vi "ezAFM Practice 1.5.vi"() -> ()   [LabVIEW 2015]
uses:
  D:/LabVIEW for ezAFM/LV-PGC 2019-05a/Special Equipment/ezAFM/NMI Integration Code/ezCommander.dll
  LabVIEW for ezAFM/LV-PGC 2019-05a/Special Equipment/ezAFM/NMI Integration Code/ezCommander.dll
  <vilib>/userdefined/High Color/IMAQdx.ctl
  LabVIEW for ezAFM/LV-PGC 2019-05a/Universal vi's/Global Variables/Globals-EasyAFM.vi
  Globals.vi
  <vilib>/vision/driver/NI_Vision_Acquisition_Software.lvlib
panel:
  out "Index":dbl
  out "Direction":dbl
  out "Searching":bool
  out "Crosshair Found?":bool
  in  "Search":bool
  out "Total Steps":dbl
  out "Current Steps":dbl
  in  "Camera":enum32{"ezAFM Camera"}(tab)
  out "ezAFM Camera":T1(plugin-control)
  out "Currently Scanning":string
  in  "Enable Automatic Repositioning?":bool
  in  "Main Menu":enum32{"Navigation", "Scanning"}(tab)
  in  "APPROACH":bool
  in  "RETRACT":bool
  in  "Step Size":dbl
  out "Angle":dbl
  in  "THETA":bool
  in  "MOVE2CROSSHAIR":bool
  in  "Current Crosshair":string(combo)="00 | 01"
  in  "Target Crosshair":string(combo)="00 | 01"
  in  "Motor Speed":u16(ring)=30000 items=["SLOW"=3300, "MEDIUM"=30000, "FAST"=65000]
  in  "Navigation Buttons":T2
  in  "SEARCH":bool
  in  "Image Resolution":u16(ring)=256 items=["32"=32, "64"=64, "128"=128, "256"=256, "512"=512, "1024"=1024, "2048"=2048]
  in  "SELECT CONNECTIONS":bool
  in  "BEGIN AUTOMATED IMAGING":bool
  out "Connections":string[](array[string])
  in  "Indicators":enum32{"Indicators"}(tab)
  out "XYZ Motor Position":dbl[](array[numeric]) format="%#_4f"
  out "ezAFM Status":dbl
  out "Approaching":bool
  out "ezAFM Connected":bool
  out "Retracting":bool
  out "Scanning":bool
  out "Tip Approached?":bool
  in  "RESET":bool
  out "XY Position":dbl[](array[numeric])
  in  "QUIT":bool
  # "Use Arrow Keys to manually\nmove the XY Motor"
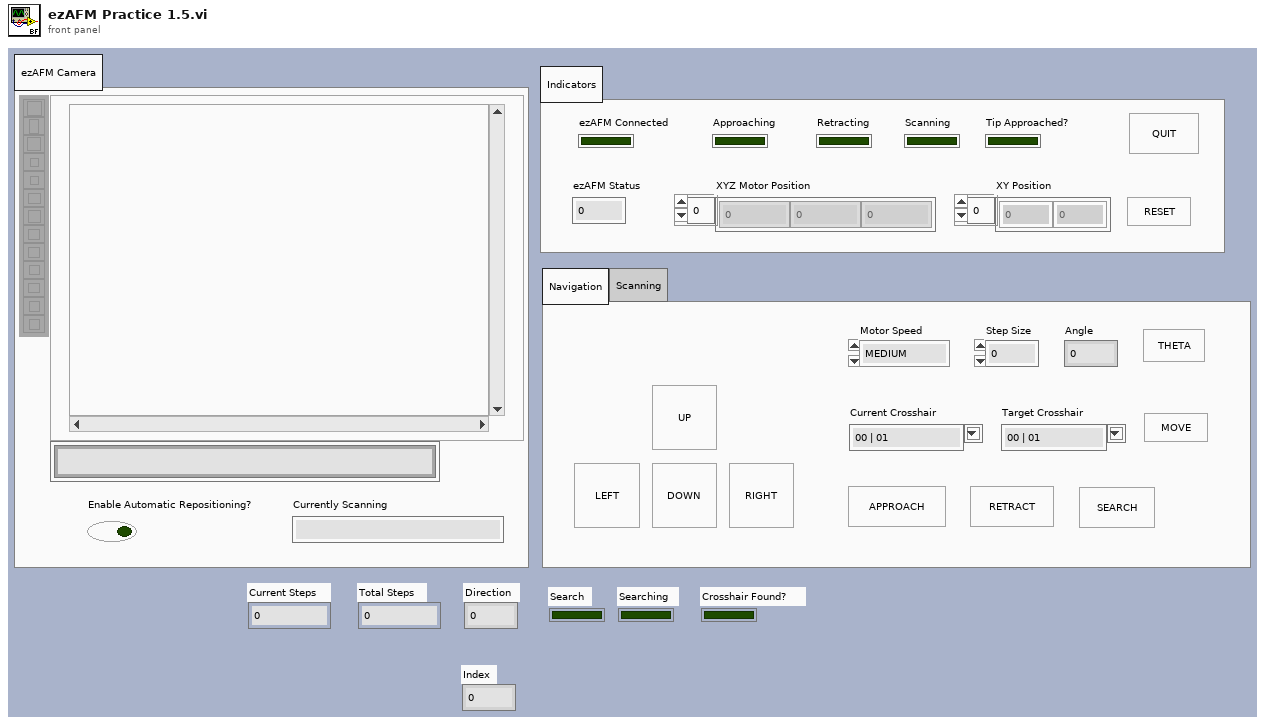
[diagram p1: front panel]
types:
  T1 = typedef "IMAQ Image.ctl" = refnum<image>
  T2 = cluster{"UP":bool, "DOWN":bool, "LEFT":bool, "RIGHT":bool}
  T3 = typedef "IMAQdx.ctl" = refnum<k21>
  T4 = typedef "Image Type" = u32
  T5 = typedef "eventvkey.ctl" = enum16{"ASCII", "Enter", "Return", "Shift", "Ctrl", "Alt", "Cmd", "Opt", "Caps", "NumLock", "Clear", "Break", "Up", "Down", "Left", "Right", "Insert", "Delete", "Home", "End", "PageUp", "PageDown", "Escape", "Help", "Pause", "ScrollLock", "F1", "F2", "F3", "F4", "F5", "F6", "F7", "F8", "F9", "F10", "F11", "F12", "F13", "F14", "F15", "F16", "F17", "F18", "F19", "F20", "F21", "F22", "F23", "F24", "Play", "VolumeUp", "VolumeDown", "Mute", "Two Byte Char"}
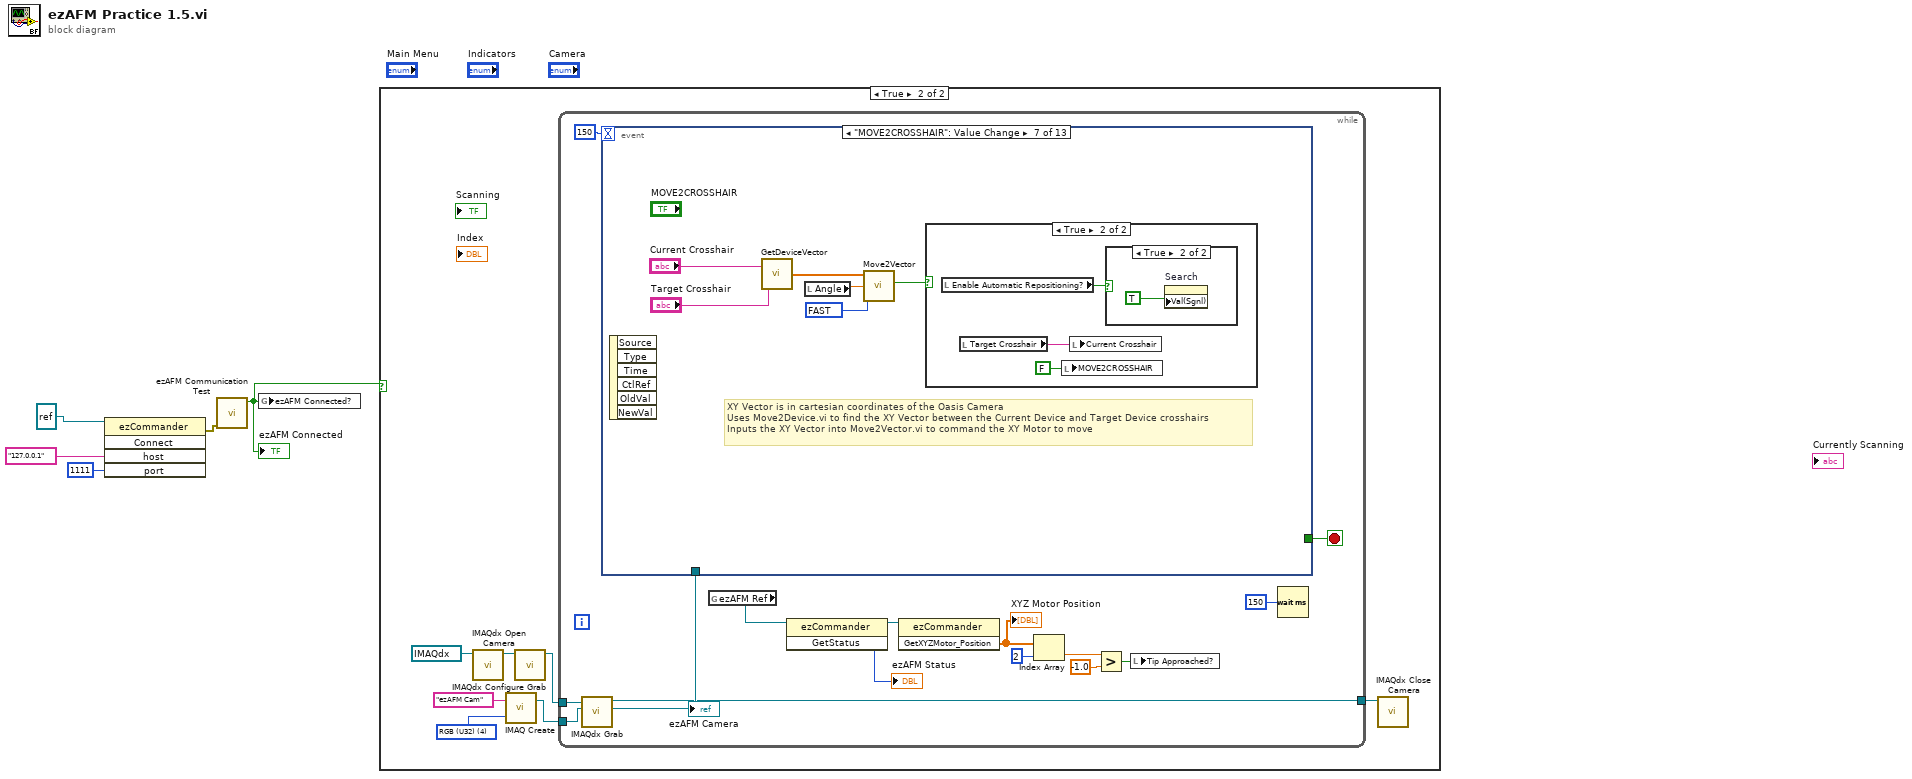
[diagram p0: block diagram]
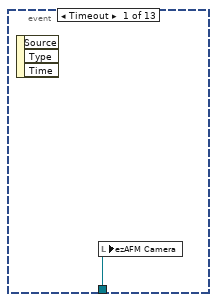
[diagram p3: hidden frame]
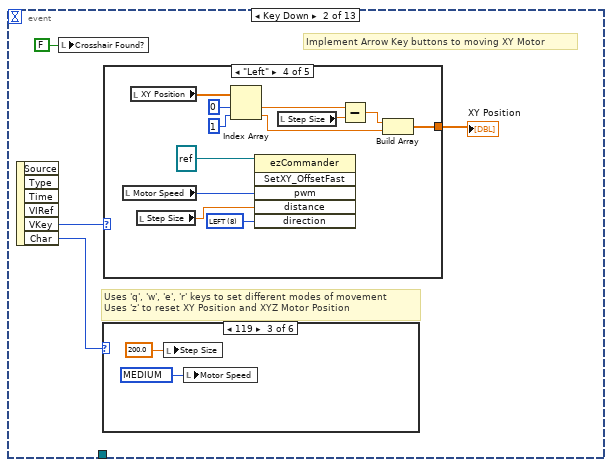
[diagram p4: hidden frame]
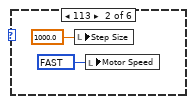
[diagram p6: hidden frame]
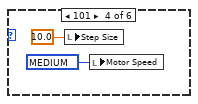
[diagram p7: hidden frame]
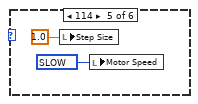
[diagram p8: hidden frame]
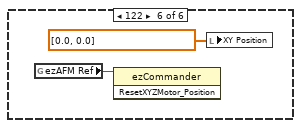
[diagram p9: hidden frame]
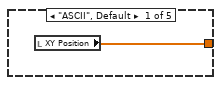
[diagram p10: hidden frame]
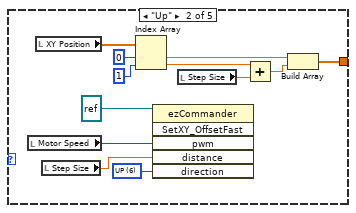
[diagram p11: hidden frame]
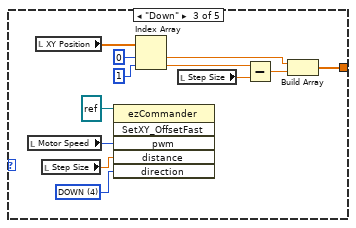
[diagram p12: hidden frame]
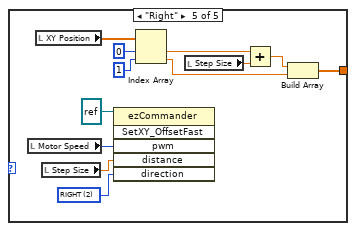
[diagram p13: hidden frame]
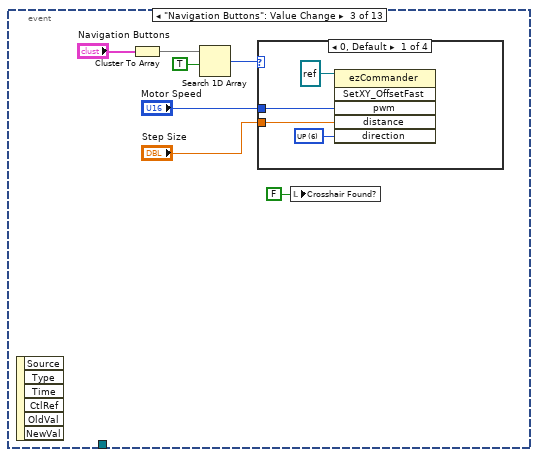
[diagram p14: hidden frame]
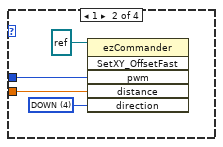
[diagram p15: hidden frame]
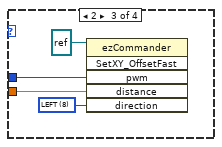
[diagram p16: hidden frame]
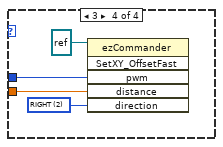
[diagram p17: hidden frame]
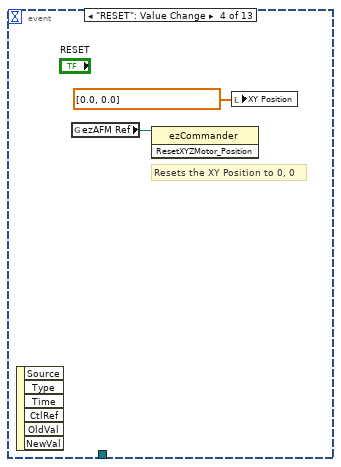
[diagram p18: hidden frame]
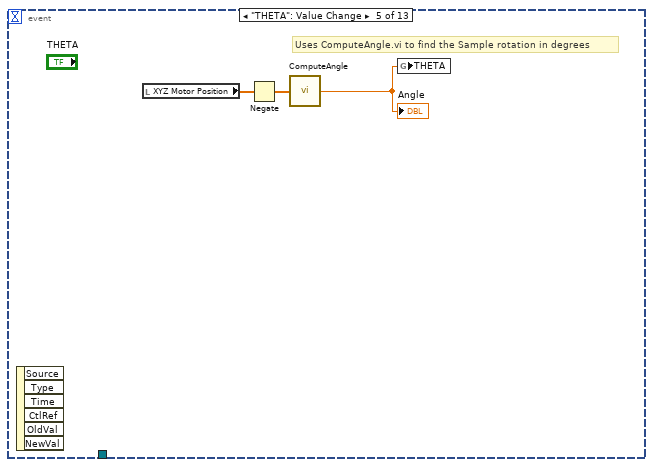
[diagram p19: hidden frame]
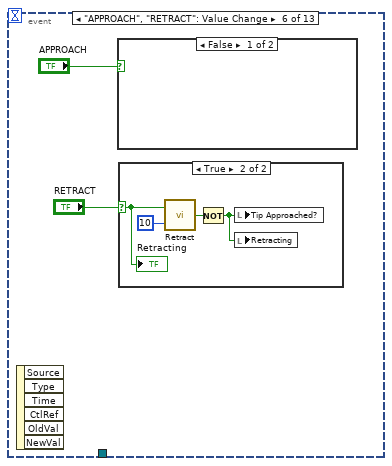
[diagram p20: hidden frame]
diagram:
  n1 = invoke class="ezCommander" method="Connect"(reference=refnum<k24> refnum ("ezAFM Ref"), "host"="127.0.0.1", "port"=1111) -> (error out=w4:errorcluster)  [unwired: 2 in, 4 out]
  n2 = call "ezAFM Communication Test.vi"("error in"=w4) -> ("ezAFM COM status"=w1:bool)  [unwired: 3 in, 3 out]
  "ezAFM Connected" <- w1
  n3 = global write "Globals.vi" "ezAFM Connected?"(w1) -> ()
  n4 = case shown="True" w1 {
    frame False {
    }
    frame True {
      w8 = T4 4 items=["Grayscale (U8)", "Grayscale (I16)", "Grayscale (SGL)", "Complex (CSG)", "RGB (U32)", "HSL (U32)", "RGB (U64)", "Grayscale (U16)"] ("Image Type")
      n5 = call <vilib>:"IMAQdx Open Camera.vi"("Session In"=T3 "cam5") -> ("Session Out"=w10:T3)  [unwired: 9 in, 1 out]
      n6 = call "IMAQ Create"("Image Name"="ezAFM Cam", "Image Type"=w8) -> ("New Image"=w9:T1)  [unwired: 3 in, 1 out]
      n7 = call <vilib>:"IMAQdx Configure Grab.vi"("Session In"=w10) -> ("Session Out"=w7:T3)  [unwired: 9 in, 1 out]
      n8 = while {
        tunnel: w9 -> [w26]
        tunnel: w7 -> [w25]
        tunnel: [w15] -> w6
        stop <- w14 stop-if-true
        n9 = call <vilib>:"IMAQdx Grab.vi"("Image In"=w26, "Session In"=w25) -> ("Image Out"=w16:T1, "Session Out"=w15:T3)  [unwired: 2 in, 6 out]
        "ezAFM Camera" <- w16
        n10 = event shown="[6] \"MOVE2CROSSHAIR\": Value Change" {
          selector: _ -> [_ _ _ _ _ _ _ _ _ _ _ _ _]
          dyn-events: _ -> [_ _ _ _ _ _ _ _ _ _ _ _ _]
          timeout: 150 -> [_ _ _ _ _ _ _ _ _ _ _ _ _]
          tunnel: [_ _ _ _ _ _ _ _ _ _ _ _ "QUIT"] -> w14
          tunnel: w16 -> [w28 _ _ _ _ _ _ _ _ _ w173 _ _]
          event Timeout {
            n11 = event-data() -> ()  [unwired: 1 in, 3 out]
            n12 = local write "ezAFM Camera"(w28) -> ()
          }
          event Key Down {
            # "Uses 'q', 'w', 'e', 'r' keys to set different modes of movement\nUses 'z' to reset XY Position and XYZ Motor Position"
            # "Implement Arrow Key buttons to moving XY Motor"
            n13 = event-data() -> ("VKey"=w30:T5, "Char"=w31:i16)  [unwired: 1 in, 4 out]
            n14 = local write "Crosshair Found?"(FALSE ("Crosshair Found?")) -> ()
            n15 = case shown="119" w31 {
              frame 0, Default {
              }
              frame 113 {
                w33 = u16 65000 items=["SLOW"=3300, "MEDIUM"=30000, "FAST"=65000] ("Motor Speed")
                n16 = local write "Step Size"(1000.0 ("Step Size")) -> ()
                n17 = local write "Motor Speed"(w33) -> ()
              }
              frame 119 {
                w35 = u16 30000 items=["SLOW"=3300, "MEDIUM"=30000, "FAST"=65000] ("Motor Speed")
                n18 = local write "Step Size"(200.0 ("Step Size")) -> ()
                n19 = local write "Motor Speed"(w35) -> ()
              }
              frame 101 {
                w37 = u16 30000 items=["SLOW"=3300, "MEDIUM"=30000, "FAST"=65000] ("Motor Speed")
                n20 = local write "Step Size"(10.0 ("Step Size")) -> ()
                n21 = local write "Motor Speed"(w37) -> ()
              }
              frame 114 {
                w39 = u16 3300 items=["SLOW"=3300, "MEDIUM"=30000, "FAST"=65000] ("Motor Speed")
                n22 = local write "Step Size"(1.0 ("Step Size")) -> ()
                n23 = local write "Motor Speed"(w39) -> ()
              }
              frame 122 {
                n24 = global read "Globals-EasyAFM.vi" "ezAFM Ref"() -> (w41:refnum<k24>)
                n25 = invoke class="ezCommander" method="ResetXYZMotor_Position"(reference=w41) -> ()  [unwired: 2 in, 3 out]
                n26 = local write "XY Position"(dbl[] [0.0, 0.0] ("XY Position")) -> ()
              }
            }
            n27 = case shown="\"Left\"" w30 {
              tunnel: [w43 w45 w56 w68 w80] -> w32
              frame "ASCII", Default {
                n28 = local read "XY Position"() -> (w43:dbl[])
              }
              frame "Up" {
                w54 = u16 6 items=["UP"=6, "DOWN"=4, "LEFT"=8, "RIGHT"=2]
                n29 = local read "Motor Speed"() -> (w53:u16)
                n30 = local read "XY Position"() -> (w51:dbl[])
                n31 = local read "Step Size"() -> (w52:dbl)
                n32 = Index Array(array=w51, index #1=0 ("index"), index #2=1 ("index")) -> (element #1=w47:dbl, element #2=w44:dbl)
                n33 = invoke class="ezCommander" method="SetXY_OffsetFast"(reference=refnum<k24> refnum ("ezAFM Ref"), "pwm"=w53, "distance"=w52, "direction"=w54) -> ()  [unwired: 2 in, 6 out]
                n34 = local read "Step Size"() -> (w48:dbl)
                n35 = Add(x=w44, y=w48) -> (x+y=w46:dbl)
                n36 = Build Array(w47, w46) -> (w45:dbl[])
              }
              frame "Down" {
                w64 = u16 4 items=["UP"=6, "DOWN"=4, "LEFT"=8, "RIGHT"=2]
                n37 = local read "Motor Speed"() -> (w66:u16)
                n38 = local read "XY Position"() -> (w58:dbl[])
                n39 = local read "Step Size"() -> (w65:dbl)
                n40 = invoke class="ezCommander" method="SetXY_OffsetFast"(reference=refnum<k24> refnum ("ezAFM Ref"), "pwm"=w66, "distance"=w65, "direction"=w64) -> ()  [unwired: 2 in, 6 out]
                n41 = Index Array(array=w58, index #1=0 ("index"), index #2=1 ("index")) -> (element #1=w60:dbl, element #2=w61:dbl)
                n42 = local read "Step Size"() -> (w57:dbl)
                n43 = Subtract(x=w61, y=w57) -> (x-y=w59:dbl)
                n44 = Build Array(w60, w59) -> (w56:dbl[])
              }
              frame "Left" {
                w78 = u16 8 items=["UP"=6, "DOWN"=4, "LEFT"=8, "RIGHT"=2]
                n45 = local read "Motor Speed"() -> (w76:u16)
                n46 = local read "XY Position"() -> (w72:dbl[])
                n47 = local read "Step Size"() -> (w77:dbl)
                n48 = Index Array(array=w72, index #1=0 ("index"), index #2=1 ("index")) -> (element #1=w71:dbl, element #2=w69:dbl)
                n49 = invoke class="ezCommander" method="SetXY_OffsetFast"(reference=refnum<k24> refnum ("ezAFM Ref"), "pwm"=w76, "distance"=w77, "direction"=w78) -> ()  [unwired: 2 in, 6 out]
                n50 = local read "Step Size"() -> (w73:dbl)
                n51 = Subtract(x=w71, y=w73) -> (x-y=w70:dbl)
                n52 = Build Array(w70, w69) -> (w68:dbl[])
              }
              frame "Right" {
                w90 = u16 2 items=["UP"=6, "DOWN"=4, "LEFT"=8, "RIGHT"=2]
                n53 = local read "Motor Speed"() -> (w89:u16)
                n54 = local read "XY Position"() -> (w85:dbl[])
                n55 = local read "Step Size"() -> (w88:dbl)
                n56 = invoke class="ezCommander" method="SetXY_OffsetFast"(reference=refnum<k24> refnum ("ezAFM Ref"), "pwm"=w89, "distance"=w88, "direction"=w90) -> ()  [unwired: 2 in, 6 out]
                n57 = Index Array(array=w85, index #1=0 ("index"), index #2=1 ("index")) -> (element #1=w83:dbl, element #2=w81:dbl)
                n58 = local read "Step Size"() -> (w84:dbl)
                n59 = Add(x=w83, y=w84) -> (x+y=w82:dbl)
                n60 = Build Array(w82, w81) -> (w80:dbl[])
              }
            }
            "XY Position" <- w32
          }
          event "Navigation Buttons": Value Change {
            n61 = event-data() -> ()  [unwired: 1 in, 6 out]
            n62 = Cluster To Array(cluster="Navigation Buttons") -> (array=w97:bool[])
            n63 = Search 1D Array(1D array=w97, element=TRUE) -> (index of element=w95:i32)  [unwired: 1 in]
            n64 = case shown="0, Default" w95 {
              tunnel: "Step Size" -> [w99 w104 w108 w112]
              tunnel: "Motor Speed" -> [w100 w103 w107 w111]
              frame 0, Default {
                w101 = u16 6 items=["UP"=6, "DOWN"=4, "LEFT"=8, "RIGHT"=2]
                n65 = invoke class="ezCommander" method="SetXY_OffsetFast"(reference=refnum<k24> refnum ("ezAFM Ref"), "pwm"=w100, "distance"=w99, "direction"=w101) -> ()  [unwired: 2 in, 6 out]
              }
              frame 1 {
                w105 = u16 4 items=["UP"=6, "DOWN"=4, "LEFT"=8, "RIGHT"=2]
                n66 = invoke class="ezCommander" method="SetXY_OffsetFast"(reference=refnum<k24> refnum ("ezAFM Ref"), "pwm"=w103, "distance"=w104, "direction"=w105) -> ()  [unwired: 2 in, 6 out]
              }
              frame 2 {
                w109 = u16 8 items=["UP"=6, "DOWN"=4, "LEFT"=8, "RIGHT"=2]
                n67 = invoke class="ezCommander" method="SetXY_OffsetFast"(reference=refnum<k24> refnum ("ezAFM Ref"), "pwm"=w107, "distance"=w108, "direction"=w109) -> ()  [unwired: 2 in, 6 out]
              }
              frame 3 {
                w113 = u16 2 items=["UP"=6, "DOWN"=4, "LEFT"=8, "RIGHT"=2]
                n68 = invoke class="ezCommander" method="SetXY_OffsetFast"(reference=refnum<k24> refnum ("ezAFM Ref"), "pwm"=w111, "distance"=w112, "direction"=w113) -> ()  [unwired: 2 in, 6 out]
              }
            }
            n69 = local write "Crosshair Found?"(FALSE ("Crosshair Found?")) -> ()
          }
          event "RESET": Value Change {
            # "Resets the XY Position to 0, 0"
            n70 = event-data() -> ()  [unwired: 1 in, 6 out]
            n71 = global read "Globals-EasyAFM.vi" "ezAFM Ref"() -> (w115:refnum<k24>)
            n72 = invoke class="ezCommander" method="ResetXYZMotor_Position"(reference=w115) -> ()  [unwired: 2 in, 3 out]
            n73 = local write "XY Position"(dbl[] [0.0, 0.0] ("XY Position")) -> ()
          }
          event "THETA": Value Change {
            # "Uses ComputeAngle.vi to find the Sample rotation in degrees"
            n74 = event-data() -> ()  [unwired: 1 in, 6 out]
            n75 = local read "XYZ Motor Position"() -> (w117:dbl[])
            n76 = Negate(x=w117) -> (-x=w118:dbl[])
            n77 = call "ComputeAngle.vi"("XY Vector"=w118) -> ("Angle"=w119:dbl)
            "Angle" <- w119
            n78 = global write "Globals.vi" "THETA"(w119) -> ()
          }
          event "APPROACH", "RETRACT": Value Change {
            n79 = event-data() -> ()  [unwired: 1 in, 6 out]
            n80 = case shown="False" "APPROACH" {
              selector: "APPROACH" -> [_ w127]
              frame False {
              }
              frame True {
                n81 = call "AutoLand&Approach.vi"("Approaching?"=w127) -> ("Finished?"=w126:bool)
                "Tip Approached?" <- w126
                n82 = Not(x=w126) -> (.not. x?=w128:bool)
                n83 = local write "Approaching"(w128) -> ()
                "Approaching" <- w127
              }
            }
            n84 = case shown="True" "RETRACT" {
              selector: "RETRACT" -> [_ w122]
              frame False {
              }
              frame True {
                n85 = call "Retract.vi"("Number of Cycles"=10, "Retracting?"=w122) -> ("Finished?"=w124:bool)
                n86 = Not(x=w124) -> (.not. x?=w123:bool)
                n87 = local write "Tip Approached?"(w123) -> ()
                n88 = local write "Retracting"(w123) -> ()
                "Retracting" <- w122
              }
            }
          }
          event "MOVE2CROSSHAIR": Value Change {
            w133 = u16 65000 items=["SLOW"=3300, "MEDIUM"=30000, "FAST"=65000] ("Motor Speed")
            # "XY Vector is in cartesian coordinates of the Oasis Camera\nUses Move2Device.vi to find the XY Vector between the Current Device and Target Device crosshairs\nInputs the XY Vector into Move2Vector.vi to command the XY Motor to move"
            n89 = event-data() -> ()  [unwired: 1 in, 6 out]
            n90 = call "GetDeviceVector.vi"("Target Device"="Target Crosshair", "Current Device"="Current Crosshair") -> ("XY Vector"=w134:dbl[])
            n91 = local read "Angle"() -> (w132:dbl)
            n92 = call "Move2Vector.vi"("Motor Speed"=w133, "Angle"=w132, "XY Vector"=w134) -> ("Finished?"=w129:bool)  [unwired: 8 in]
            n93 = case shown="True" w129 {
              frame False {
              }
              frame True {
                n94 = local read "Enable Automatic Repositioning?"() -> (w137:bool)
                n95 = local read "Target Crosshair"() -> (w136:string)
                n96 = local write "MOVE2CROSSHAIR"(FALSE) -> ()
                n97 = local write "Current Crosshair"(w136) -> ()
                n98 = case shown="True" w137 {
                  frame False {
                  }
                  frame True {
                    n99 = property on="Search" class="Bool (strict)"("Val(Sgnl)"=TRUE ("Value (Signaling)")) -> ()  [unwired: 2 in, 2 out]
                  }
                }
              }
            }
          }
          event "SELECT CONNECTIONS": Value Change {
            n100 = event-data() -> ()  [unwired: 1 in, 6 out]
            n101 = case shown="True" "SELECT CONNECTIONS" {
              frame False {
              }
              frame True {
                n102 = call "SelectConnections.vi"() -> ("Selected Connections"=→"Connections":string[])  [unwired: 1 in]
              }
            }
          }
          event "Enable Automatic Repositioning?": Value Change {
            w141 = u16 6 items=["UP"=6, "DOWN"=4, "LEFT"=8, "RIGHT"=2]
            n103 = event-data() -> ()  [unwired: 1 in, 6 out]
            "Total Steps" <- 1.0 ("Total Distance")
            "Current Steps" <- 0.0 ("Current Steps")
            "Direction" <- w141
          }
          event "BEGIN AUTOMATED IMAGING": Value Change {
            n104 = event-data() -> ("NewVal"=w144:bool)  [unwired: 1 in, 5 out]
            n105 = local read "Connections"() -> (w147:string[])
            n106 = local write "Enable Automatic Repositioning?"(w144) -> ()
            n107 = call "BuildSequence.vi"("Connections"=w147) -> ("Sequence"=w146:string[])
            n108 = for {
              tunnel: w146 -> [w149] mode=indexing
              tunnel: "Image Resolution" -> [w148]
              n109 = Search/Split String(string=w149, search string/char (-)="Scan Spot") -> (offset of match=w152:i32)  [unwired: 1 in, 2 out]
              n110 = Search/Split String(string=w149, search string/char (-)="Crosshairs") -> (offset of match=w153:i32)  [unwired: 1 in, 2 out]
              n111 = Greater Or Equal To 0?(x=w152) -> (x >= 0?=w151:bool)
              n112 = Greater Or Equal To 0?(x=w153) -> (x >= 0?=w150:bool)
              n113 = case shown="True" w150 {
                tunnel: w149 -> [_ w160]
                frame False {
                }
                frame True {
                  n114 = String Subset(string=w160, offset (0)=21, length (rest)=7 ("length (rest)")) -> (substring=w158:string)
                  n115 = String Subset(string=w160, offset (0)=10, length (rest)=7 ("length (rest)")) -> (substring=w159:string)
                  n116 = local write "Target Crosshair"(w158) -> ()
                  n117 = local write "Current Crosshair"(w159) -> ()
                  n118 = String Length(string=w158) -> (length=w157:i32)
                  n119 = Greater Than 0?(x=w157) -> (x > 0?=w156:bool)
                  n120 = property on="MOVE2CROSSHAIR" class="Bool (strict)"("Val(Sgnl)"=w156) -> ()  [unwired: 2 in, 2 out]
                }
              }
              n121 = case shown="True" w151 {
                tunnel: w149 -> [_ w169]
                tunnel: w148 -> [_ w166]
                frame False {
                }
                frame True {
                  n122 = String Subset(string=w169, offset (0)=17) -> (substring=w167:string)  [unwired: 1 in]
                  n123 = local read "Angle"() -> (w165:dbl)
                  n124 = call "TakeScan.vi"("Angle"=w165, "Image Resolution"=w166, "Scan Spot"=w167, "Connection"=w169) -> ()  [unwired: 7 in, 1 out]
                }
              }
            }
          }
          event "SEARCH", "Search": Value Change {
            n125 = event-data() -> ("NewVal"=w170:bool)  [unwired: 1 in, 5 out]
            n126 = while {
              tunnel: w173 -> [w180]
              tunnel: [w176] -> w171
              tunnel: [w179] -> w172
              i -> [w177]
              stop <- w174 stop-if-true
              n127 = Greater?(x=w177, y=5.0) -> (0:w175:bool)
              n128 = call "IdentifyCrosshair.vi"("ezAFM Camera"=w180) -> ("Delta"=w179:dbl[], "Found?"=w176:bool)
              n129 = Or(x=w175, y=w176) -> (x .or. y?=w174:bool)
            }
            "Crosshair Found?" <- w171
            n130 = local write "Searching"(w170) -> ()
            n131 = case shown="False" w171 {
              selector: w171 -> [w181 _]
              tunnel: w172 -> [_ w187]
              frame False {
                n132 = local write "Searching"(w181) -> ()
                n133 = local read "Enable Automatic Repositioning?"() -> (w182:bool)
                n134 = case shown="True" w182 {
                  frame False {
                  }
                  frame True {
                    n135 = property on="Searching" class="Bool (strict)"("Val(Sgnl)"=TRUE ("Value (Signaling)")) -> ()  [unwired: 2 in, 2 out]
                  }
                }
              }
              frame True {
                w184 = FALSE ("SEARCH")
                w186 = u16 3300 items=["SLOW"=3300, "MEDIUM"=30000, "FAST"=65000] ("Motor Speed")
                n136 = local write "Searching"(w184) -> ()
                n137 = local write "Search"(w184) -> ()
                n138 = call "Move2Vector.vi"("Motor Speed"=w186, "Angle"=0.0, "XY Vector"=w187) -> ()  [unwired: 8 in, 1 out]
              }
            }
          }
          event "Searching": Value Change {
            n139 = event-data() -> ()  [unwired: 1 in, 6 out]
            n140 = local read "Total Steps"() -> (w188:dbl)
            n141 = local read "Current Steps"() -> (w190:dbl)
            n142 = local read "Direction"() -> (w191:dbl)
            n143 = property on="Search" class="Bool (strict)"("Val(Sgnl)"=TRUE ("Value (Signaling)")) -> ()  [unwired: 2 in, 2 out]
            n144 = Equal?(x=w188, y=w190) -> (x = y?=w192:bool)
            n145 = case shown="True" w192 {
              tunnel: w190 -> [w194 _]
              tunnel: w191 -> [w195 w201]
              tunnel: w188 -> [_ w200]
              frame False {
                w196 = u16 30000 items=["SLOW"=3300, "MEDIUM"=30000, "FAST"=65000] ("Motor Speed")
                n146 = Increment(x=w194) -> (x+1=w193:dbl)
                n147 = local write "Current Steps"(w193) -> ()
                n148 = invoke class="ezCommander" method="SetXY_OffsetFast"(reference=refnum<k24> refnum ("ezAFM Ref"), "pwm"=w196, "distance"=10.0, "direction"=w195) -> ()  [unwired: 2 in, 6 out]
              }
              frame True {
                n149 = case shown="6" w201 {
                  tunnel: [u16 0 w206 w207 w208 w209] -> w199
                  frame Default {
                  }
                  frame 6 {
                    w206 = u16 2 items=["UP"=6, "DOWN"=4, "LEFT"=8, "RIGHT"=2]
                  }
                  frame 4 {
                    w207 = u16 8 items=["UP"=6, "DOWN"=4, "LEFT"=8, "RIGHT"=2]
                  }
                  frame 8 {
                    w208 = u16 6 items=["UP"=6, "DOWN"=4, "LEFT"=8, "RIGHT"=2]
                  }
                  frame 2 {
                    w209 = u16 4 items=["UP"=6, "DOWN"=4, "LEFT"=8, "RIGHT"=2]
                  }
                }
                n150 = local write "Current Steps"(0.0 ("Current Steps")) -> ()
                n151 = local write "Direction"(w199) -> ()
                n152 = case shown="6" w199 {
                  tunnel: w200 -> [_ w203]
                  frame Default {
                  }
                  frame 6 {
                    n153 = Increment(x=w203) -> (x+1=w204:dbl)
                    n154 = local write "Total Steps"(w204) -> ()
                  }
                }
              }
            }
          }
          event "QUIT": Value Change {
            w210 = FALSE ("ezAFM Connected?")
            n155 = event-data() -> ()  [unwired: 1 in, 6 out]
            n156 = global write "Globals.vi" "ezAFM Connected?"(w210) -> ()
            n157 = local write "ezAFM Connected"(w210) -> ()
          }
        }
        n158 = global read "Globals-EasyAFM.vi" "ezAFM Ref"() -> (w17:refnum<k24>)
        n159 = invoke class="ezCommander" method="GetStatus"(reference=w17) -> (reference out=w19:refnum<k24>, "GetStatus"=→"ezAFM Status":i32)  [unwired: 2 in, 1 out]
        n160 = invoke class="ezCommander" method="GetXYZMotor_Position"(reference=w19) -> ("GetXYZMotor_Position"=w20:dbl[])  [unwired: 2 in, 2 out]
        "XYZ Motor Position" <- w20
        n161 = Index Array(array=w20, index=2) -> (element=w21:dbl)
        n162 = Greater?(x=w21, y=-1.0) -> (0:w13:bool)
        n163 = local write "Tip Approached?"(w13) -> ()
        n164 = Wait (ms)(milliseconds to wait=u32 150) -> ()  [unwired: 1 out]
      }
      n165 = call <vilib>:"IMAQdx Close Camera.vi"("Session In"=w6) -> ()  [unwired: 1 in, 10 out]
    }
  }
